vi "MC sections handling check.vi"(11 "Section name":string) -> (3 "Section is \"Initial MovCor Values\" AND MC is supported":bool)   [LabVIEW 2017]
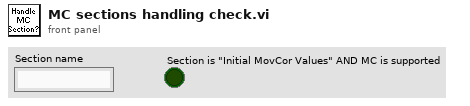
[diagram p1: front panel]
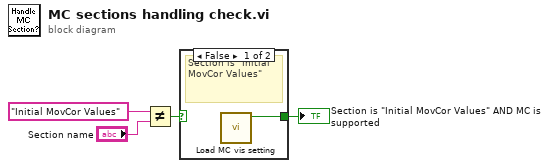
[diagram p0: block diagram]
diagram:
  n1 = Not Equal?(x="Initial MovCor Values", y="Section name") -> (x != y?=w1:bool)
  n2 = case shown="False" w1 {
    selector: w1 -> [_ w6]
    tunnel: [w5 w6] -> w4
    frame False {
      # "Section is \"Initial MovCor Values\""
      n3 = call "Load MC vis setting.vi"() -> ("MC Visible?"=w5:bool)  [unwired: 10 in, 1 out]
    }
    frame True {
      # "Any other section"
    }
  }
  "Section is \"Initial MovCor Values\" AND MC is supported" <- w4
